vi "Reset_Lockout.vi"(4 "error in (no error)":errorcluster, 5 "Boiler Simulation Controls":refnum<vi>, 6 "Boiler Controls":refnum<vi>) -> (0 "error out":errorcluster, 3 "State Out":T1)   [LabVIEW 2023]
uses:
  Controls/State.ctl
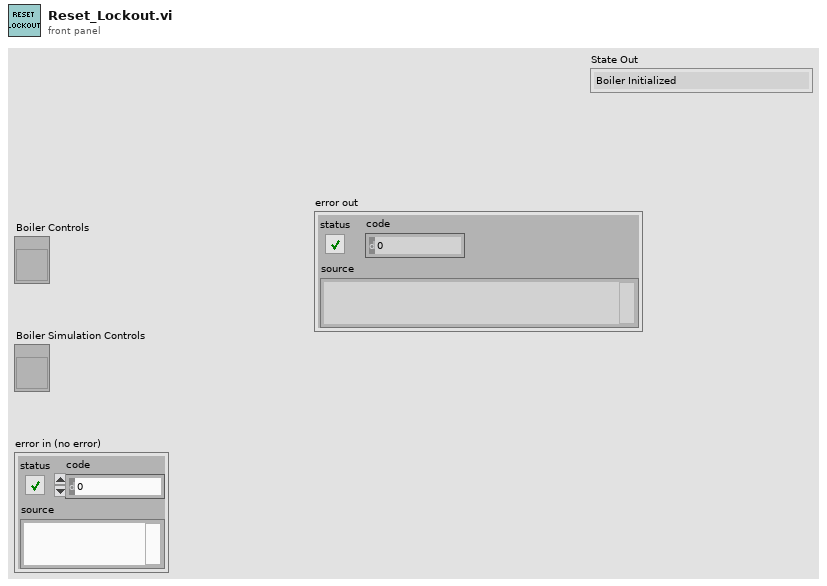
[diagram p1: front panel]
types:
  T1 = typedef "State.ctl" = enum16{"Boiler Initialized", "Boiler Ready", "Start Pre-Purge", "Pre-Purge Complete", "Pilot On", "Pilot Proved", "Force Draft Fan ON", "Shutdown and Purge", "Wait for Something"}
  T2 = typedef "Boiler Controls.ctl" = cluster{"Boiler Reset":bool, "Start Sequence":bool, "Pilot":bool, "Shutdown":bool, "Fuel Valve Position":dbl}
  T3 = typedef "Boiler Simulation Controls.ctl" = cluster{"Flame Sensor Value (%)":dbl, "Run Interlock":bool, "Forced Draft Fan":bool}
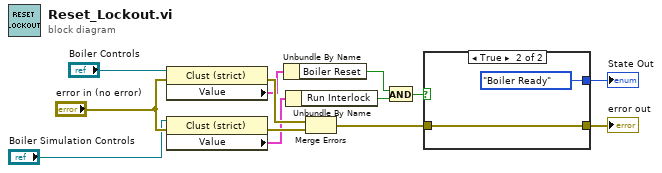
[diagram p0: block diagram]
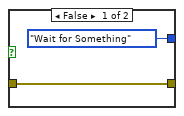
[diagram p2: hidden frame]
diagram:
  n1 = property class="Clust (strict)"(reference="Boiler Controls", error in="error in (no error)") -> (error out=w11:errorcluster, "Value"=w6:T2)  [unwired: 1 out]
  n2 = property class="Clust (strict)"(reference="Boiler Simulation Controls", error in="error in (no error)") -> (error out=w12:errorcluster, "Value"=w8:T3)  [unwired: 1 out]
  n3 = Unbundle By Name(w6) -> ("Boiler Reset"=w1:bool)
  n4 = Unbundle By Name(w8) -> ("Run Interlock"=w9:bool)
  n5 = Merge Errors(w11, w12) -> (w3:errorcluster)
  n6 = And(x=w1, y=w9) -> (x .and. y?=w13:bool)
  n7 = case shown="True" w13 {
    tunnel: [State."Wait for Something" State."Boiler Ready"] -> w4
    tunnel: w3 -> [w15 w17]
    tunnel: [w15 w17] -> w2
    frame False {
    }
    frame True {
    }
  }
  "error out" <- w2
  "State Out" <- w4
